vi "Lab2 Resistance to Colours.vi"() -> ()   [LabVIEW 2016]
panel:
  out "Resistance Measured":dbl=46600.0
  in  "Range (Ohms)":sgl(ring)=200000.0 items=["200ohm"=200, "2Kohm"=2000, "20Kohm"=20000, "200Kohm"=200000, "2Mohm"=2000000, "20Mohm"=2e+07]
  out "Band 3":u32(colorbox)=16750592
  out "Band 2":u32(colorbox)=16067327
  out "Band 1":u32(colorbox)=16776960
  in  "ResistorColours":u32[](array[colorbox])=[0, 16730368, 16711680, 16750592, 16776960, 6618880, 3381759, 16067327, 11776947, 16448250]
  # "0"
  # "1"
  # "2"
  # "3"
  # "4"
  # "5"
  # "6"
  # "7"
  # "8"
  # "9"
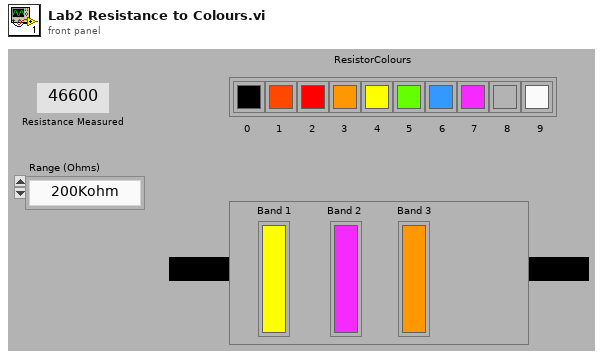
[diagram p1: front panel]
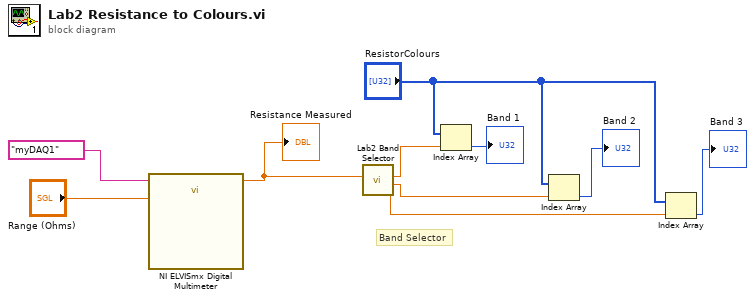
[diagram p0: block diagram]
diagram:
  # "Band Selector"
  n1 = call "NI ELVISmx Digital Multimeter"("Device Name"=tag "myDAQ1", "myDAQ Resistance Input Range (Ohms)"="Range (Ohms)") -> ("Measurement"=w4:dbl)  [unwired: 15 in, 2 out]
  "Resistance Measured" <- w4
  n2 = call "Lab2 Band Selector.vi"("resistor"=w4) -> ("band3"=w1:dbl, "band2"=w2:dbl, "band1"=w3:dbl)  [unwired: 8 in]
  n3 = Index Array(array="ResistorColours", index=w3) -> (element=→"Band 1":u32)
  n4 = Index Array(array="ResistorColours", index=w2) -> (element=→"Band 2":u32)
  n5 = Index Array(array="ResistorColours", index=w1) -> (element=→"Band 3":u32)
